vi "FPGA_fast cycles-4.vi"() -> ()   [LabVIEW 2013]
uses:
  fast cycles/FPGA_run-states.ctl
  <vilib>/rvi/Emulation/niFpgaSctlEmulationGetInTimedLoop.vi
  <vilib>/rvi/Emulation/niFpgaEmulationReportErrorSimple.vi
  <vilib>/rvi/Emulation/niFpgaGetClockAttributes.vi
  <vilib>/rvi/FIFO/Fifo_Resource/nirvififoEmulationReadFpgaImpl.vi
  <vilib>/rvi/DataTransferAndStorage/Container/Common/niFpgaContainerGetUniqueNameForEmu.vi
  <vilib>/rvi/Emulation/niFpgaProcessEmulError.vi
  <vilib>/rvi/Memory/Memory_Emulation/nirvimemoryEmulation.vi
  <vilib>/rvi/Memory/Memory_Emulation/nirvimemoryFastEmulation.vi
  <vilib>/rvi/Memory/Memory_Emulation/niFpgaMemoryEmulationCacheClearOnFirstRun.vi
  <vilib>/rvi/Memory/Memory_Emulation/nirvimemoryEmulationManagerCache_MakeExclusive.vi
  <vilib>/rvi/Memory/Memory_Emulation/niFpgaMemoryEmulationValidateCache.vi
  <vilib>/rvi/Memory/Memory_Emulation/nirvimemoryEmulationManagerCache_ReleaseExclusive.vi
  <vilib>/rvi/Memory/Memory_Emulation/nirvimemoryEmulationManagerCache_InsertValue.vi
  <vilib>/Utility/error.llb/Clear Errors.vi
  <vilib>/rvi/Memory/Memory_Emulation/nirvimemoryEmulationManagerCache_SetValue.vi
  <vilib>/rvi/Emulation/niFpgaSctlEmulationResourceMgr.vi
  <vilib>/rvi/Emulation/niFpgaCriticalErrorInLSC.vi
  <vilib>/rvi/Memory/Memory_Emulation/nirvimemoryEmulationManagerCache_GetValue.vi
  <vilib>/rvi/FIFO/Fifo_Resource/nirvififoEmulationWriteFpgaImpl.vi
  <vilib>/rvi/eio/common/nirviEmuTemplateMethod_errors.vi
  <vilib>/rvi/DataTransferAndStorage/Container/XNode/niFpgaContainer.xnode
  <vilib>/rvi/FIFO/Fifo_Resource/nirvififoEmulationRead.vi
  <vilib>/rvi/FIFO/Fifo_Resource/nirvififoEmulationWrite.vi
  <vilib>/eio/EIONode/EIONode.xnode
panel:
  out "ramp":bool
  out "trigDAC":bool
  in  "order in":u64=360850920143060992
  in  "get order":bool
  in  "Stop seq 2":bool=TRUE
  in  "stop on sample count":bool
  in  "samples":u16=1
  in  "pulse length":u16=100
  in  "Divider":u32=200000
  out "voltmeters trig":bool=TRUE
  in  "Stop seq":bool=TRUE
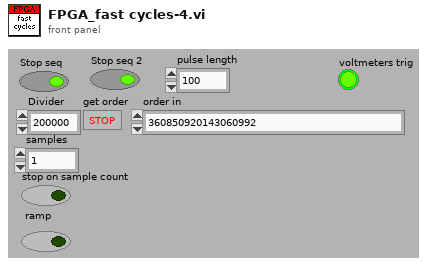
[diagram p1: front panel]
types:
  T1 = typedef "FPGA_run-states.ctl" = enum16{"stopped", "check", "reserve", "run", "release"}
  T2 = cluster{"Boolean array[0]":bool, "Boolean array[1]":bool, "Boolean array[2]":bool, "Boolean array[3]":bool, "Boolean array[4]":bool, "Boolean array[5]":bool, "Boolean array[6]":bool, "Boolean array[7]":bool, "Boolean array[8]":bool, "Boolean array[9]":bool, "Boolean array[10]":bool, "Boolean array[11]":bool, "Boolean array[12]":bool, "Boolean array[13]":bool, "Boolean array[14]":bool, "Boolean array[15]":bool}
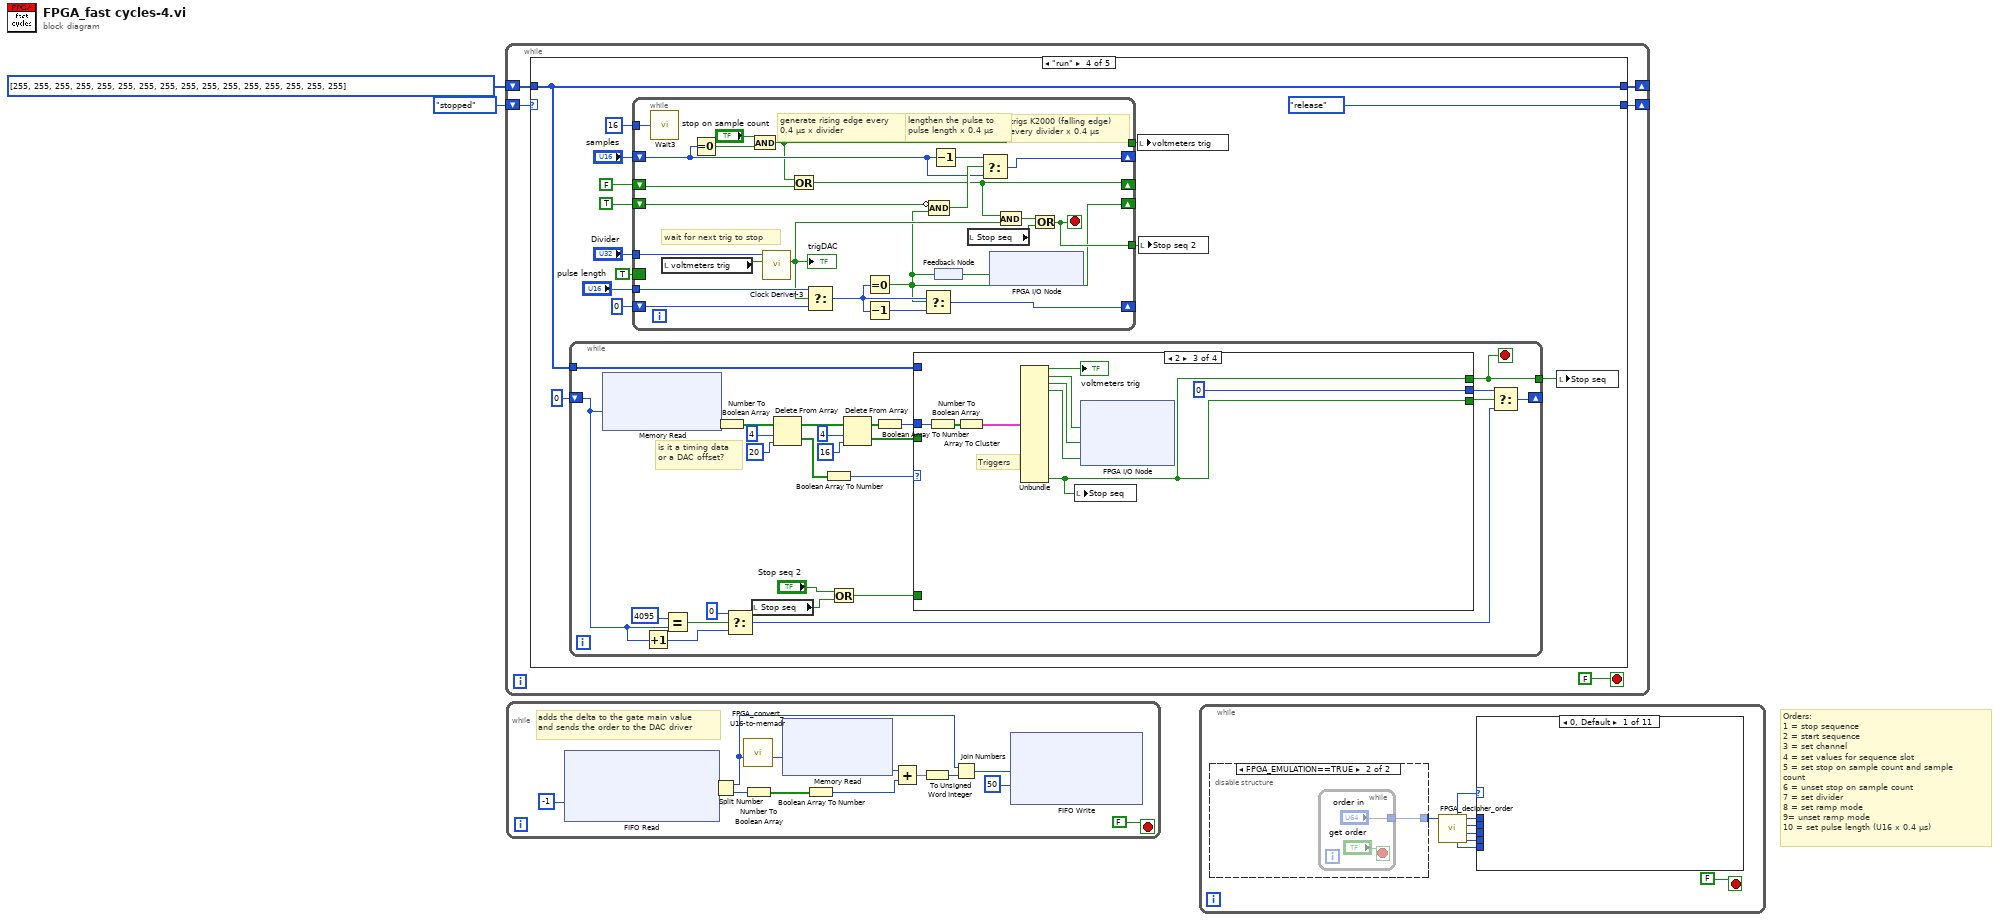
[diagram p0: block diagram]
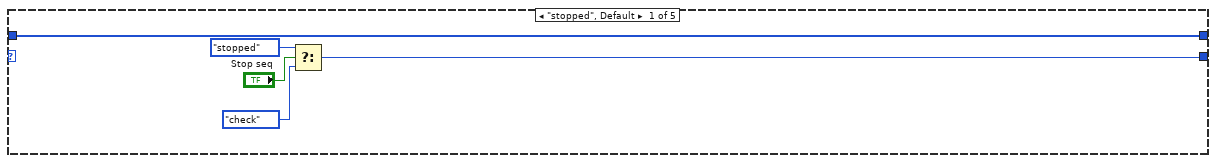
[diagram p2: hidden frame]
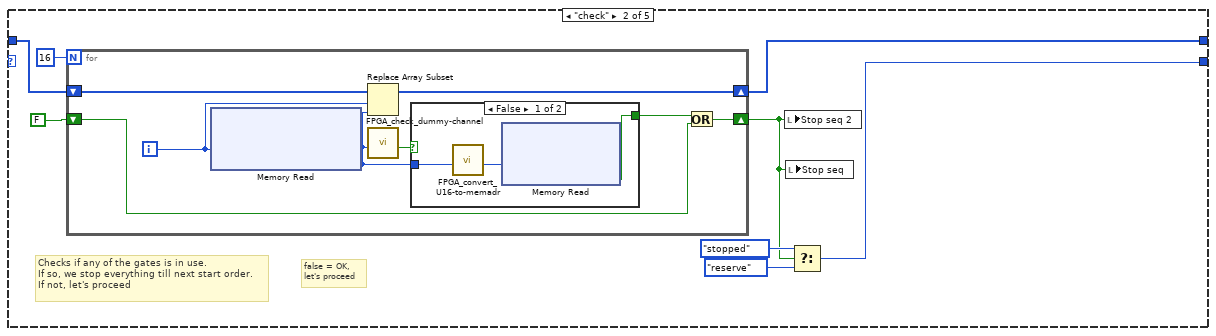
[diagram p3: hidden frame]
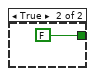
[diagram p4: hidden frame]
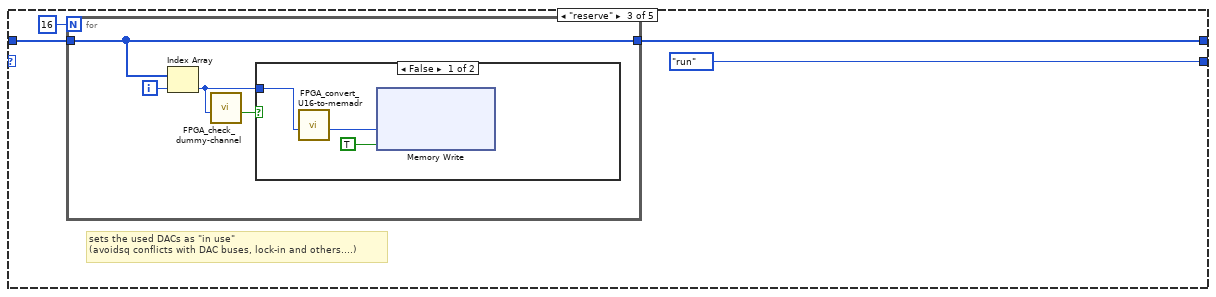
[diagram p5: hidden frame]
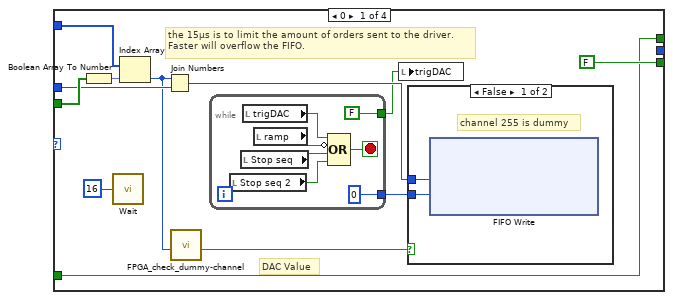
[diagram p7: hidden frame]
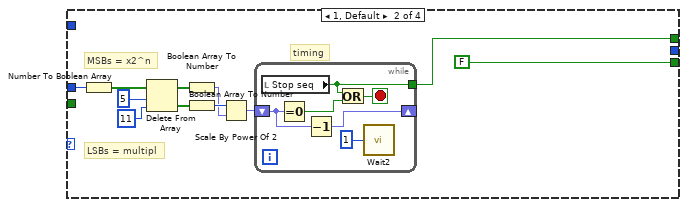
[diagram p9: hidden frame]
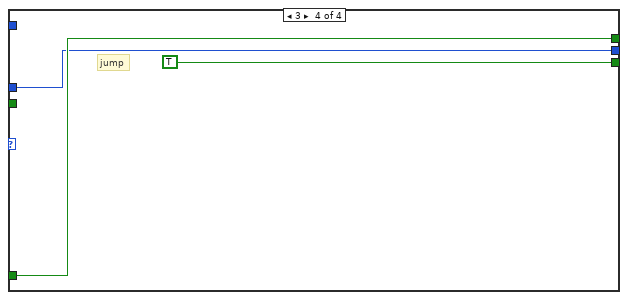
[diagram p10: hidden frame]
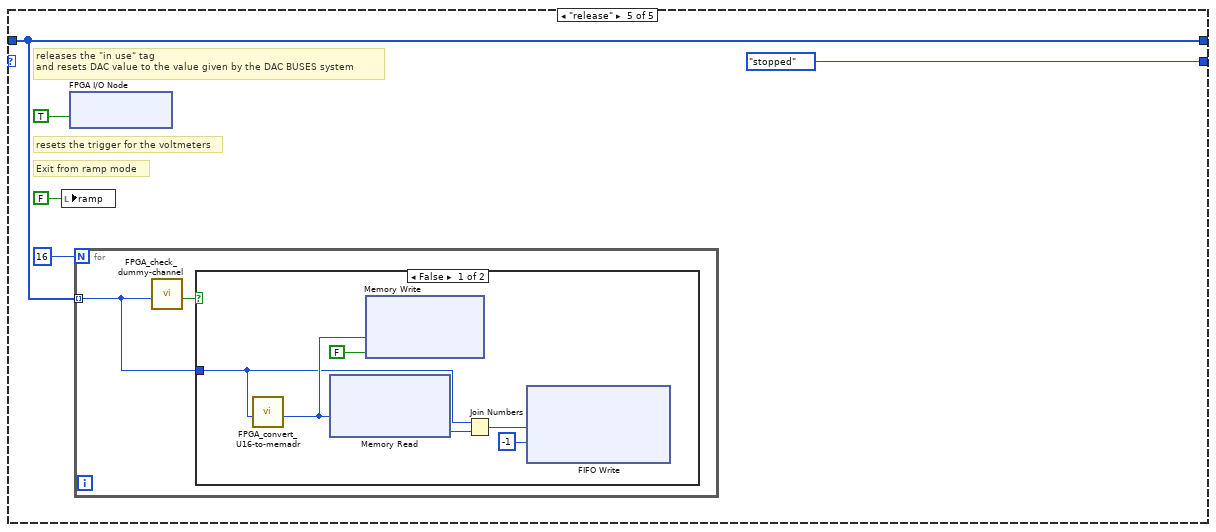
[diagram p11: hidden frame]
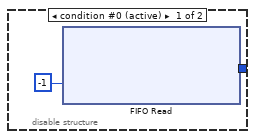
[diagram p13: hidden frame]
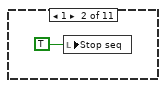
[diagram p14: hidden frame]
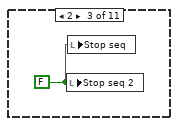
[diagram p15: hidden frame]
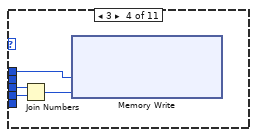
[diagram p16: hidden frame]
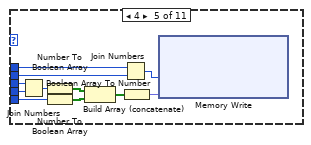
[diagram p17: hidden frame]
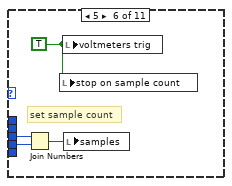
[diagram p18: hidden frame]
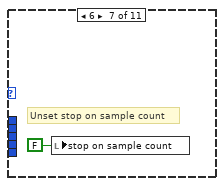
[diagram p19: hidden frame]
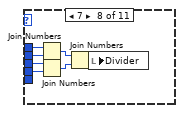
[diagram p20: hidden frame]
diagram:
  # "Orders:\n1 = stop sequence\n2 = start sequence\n3 = set channel\n4 = set values for sequence slot\n5 = set stop on sample count and sample count\n6 = unset stop on sample count\n7 = set divider\n8 = set ramp mode\n9= unset ramp mode\n10 = set pulse length (U16 x 0.4 µs)"
  n1 = while {
    shift-right: [w5] -> _
    shift-left: FPGA_run-states."stopped" ("run states") -> [w6]
    shift-right: [w3] -> _
    shift-left: u16[] [255, 255, 255, 255, 255, 255, 255, 255, 255, 255, 255, 255, 255, 255, 255, 255] -> [w4]
    stop <- FALSE stop-if-true
    n2 = case shown="\"run\"" w6 {
      tunnel: [w9 w13 FPGA_run-states."run" ("run states") FPGA_run-states."release" ("run states") FPGA_run-states."stopped" ("run states")] -> w5
      tunnel: [w8 w14 w33 w47 w159] -> w3
      tunnel: w4 -> [w8 w15 w34 w47 w159]
      frame "stopped", Default {
        n3 = Select(t=FPGA_run-states."stopped" ("run states"), s="Stop seq", f=FPGA_run-states."check" ("run states")) -> (s? t:f=w9:T1)
      }
      frame "check" {
        # "Checks if any of the gates is in use.\nIf so, we stop everything till next start order.\nIf not, let's proceed"
        # "false = OK,\nlet's proceed"
        n4 = for {
          N: 16 -> [_]
          shift-right: [w26] -> w16
          shift-left: FALSE ("Data") -> [w25]
          shift-right: [w24] -> w14
          shift-left: w15 -> [w23]
          i -> [w28]
          n5 = xnode ("Memory Read")("Address"=w28) -> ("Data"=w21:u16)  [unwired: 1 in, 1 out]
          n6 = Replace Array Subset(array=w23, new element=w21, index=w28) -> (w24:u16[])
          n7 = call "FPGA_check_dummy-channel.vi"("pan-channel"=w21) -> ("dummy?"=w22:bool)  [unwired: 10 out]
          n8 = case shown="False" w22 {
            tunnel: w21 -> [w31 _]
            tunnel: [w29 FALSE ("Data")] -> w27
            frame False {
              n9 = call "FPGA_convert_U16-to-memadr.vi"("Numeric"=w31) -> ("mem adr"=w30:u8)  [unwired: 10 out]
              n10 = xnode ("Memory Read")("Address"=w30) -> ("Data"=w29:bool)  [unwired: 1 in, 1 out]
            }
            frame True {
            }
          }
          n11 = Or(x=w27, y=w25) -> (x .or. y?=w26:bool)
        }
        n12 = local write "Stop seq 2"(w16) -> ()
        n13 = local write "Stop seq"(w16) -> ()
        n14 = Select(t=FPGA_run-states."stopped" ("run states"), s=w16, f=FPGA_run-states."reserve" ("run states")) -> (s? t:f=w13:T1)
      }
      frame "reserve" {
        # "sets the used DACs as \"in use\"\n(avoidsq conflicts with DAC buses, lock-in and others....)"
        n15 = for {
          N: 16 -> [_]
          tunnel: w34 -> [w39]
          tunnel: [w39] -> w33
          i -> [w40]
          n16 = Index Array(array=w39, index=w40) -> (element=w38:u16)
          n17 = call "FPGA_check_dummy-channel.vi"("pan-channel"=w38) -> ("dummy?"=w37:bool)  [unwired: 10 out]
          n18 = case shown="False" w37 {
            tunnel: w38 -> [w41 _]
            frame False {
              n19 = call "FPGA_convert_U16-to-memadr.vi"("Numeric"=w41) -> ("mem adr"=w43:u8)  [unwired: 10 out]
              n20 = xnode ("Memory Write")("Address"=w43, "Data"=TRUE) -> ()  [unwired: 1 in, 1 out]
            }
            frame True {
            }
          }
        }
      }
      frame "run" {
        n21 = while {
          shift-right: [w90] -> _
          shift-left: u16 0 ("t") -> [w102]
          tunnel: [w83] -> w49
          tunnel: w47 -> [w82]
          stop <- w83 stop-if-true
          # "is it a timing data\nor a DAC offset?"
          n22 = xnode ("Memory Read")("Address"=w102) -> ("Data"=w101:fxp<+,24,24>)  [unwired: 1 in, 1 out]
          n23 = Increment(x=w102) -> (x+1=w104:u16)
          n24 = Equal?(x=u16 4095, y=w102) -> (x = y?=w106:bool)
          n25 = Number To Boolean Array(number=w101) -> (Boolean array=w100:bool[])
          n26 = Select(t=u16 0, s=w106, f=w104) -> (s? t:f=w103:u16)
          n27 = local read "Stop seq"() -> (w87:bool)
          n28 = Delete From Array(array=w100, length=4, index=20) -> (deleted portion=w93:bool[], array with subset deleted=w97:bool[])
          n29 = Boolean Array To Number(Boolean array=w93) -> (number=w91:u8)
          n30 = Or(x="Stop seq 2", y=w87) -> (x .or. y?=w85:bool)
          n31 = Delete From Array(array=w97, length=4, index=16) -> (deleted portion=w94:bool[], array with subset deleted=w95:bool[])
          n32 = Boolean Array To Number(Boolean array=w95) -> (number=w86:u16)
          n33 = case shown="2" w91 {
            tunnel: w86 -> [w117 w139 w154 w155]
            tunnel: w94 -> [w119 _ _ _]
            tunnel: [FALSE ("Stop seq") FALSE ("Stop seq") w148 TRUE ("Stop seq")] -> w89
            tunnel: [_ _ u16 0 w155] -> w88
            tunnel: [w113 w129 w148 w156] -> w83
            tunnel: w85 -> [w113 _ _ w156]
            tunnel: w82 -> [w111 _ _ _]
            frame 0 {
              # "the 15µs is to limit the amount of orders sent to the driver.\nFaster will overflow the FIFO."
              # "DAC Value"
              n34 = Boolean Array To Number(Boolean array=w119) -> (number=w118:fxp<+,4,4>)
              n35 = call "Wait"("Count(uSec)"=u8 16) -> ()  [unwired: 1 out]
              n36 = Index Array(array=w111, index=w118) -> (element=w109:u16)
              n37 = Join Numbers(hi=w109, lo=w117) -> ((hi.lo)=w116:u32)
              n38 = call "FPGA_check_dummy-channel.vi"("pan-channel"=w109) -> ("dummy?"=w110:bool)  [unwired: 10 out]
              n39 = while {
                tunnel: [0 ("Timeout")] -> w112
                tunnel: [FALSE ("Stop seq 3")] -> w108
                stop <- w123 stop-if-true
                n40 = local read "Stop seq 2"() -> (w126:bool)
                n41 = local read "Stop seq"() -> (w127:bool)
                n42 = local read "trigDAC"() -> (w124:bool)
                n43 = local read "ramp"() -> (w125:bool)
                n44 = Compound Arithmetic op=OR(w124, invert w125, w127, w126) -> (w123:bool)
              }
              n45 = local write "trigDAC"(w108) -> ()
              n46 = case shown="False" w110 {
                tunnel: w116 -> [w121 _]
                tunnel: w112 -> [w120 _]
                frame False {
                  # "channel 255 is dummy"
                  n47 = xnode ("FIFO Write")("Element"=w121, "Timeout"=w120) -> ()  [unwired: 1 in, 2 out]
                }
                frame True {
                }
              }
            }
            frame 1, Default {
              # "MSBs = x2^n"
              # "LSBs = multipl"
              # "timing"
              n48 = Number To Boolean Array(number=w139) -> (Boolean array=w138:bool[])
              n49 = Delete From Array(array=w138, length=5 ("longueur"), index=11 ("indice")) -> (deleted portion=w134:bool[], array with subset deleted=w135:bool[])
              n50 = Boolean Array To Number ("Tableau de booléens en nombre")(Boolean array=w135) -> (number=w132:fxp<+,37,37>)
              n51 = Boolean Array To Number ("Tableau de booléens en nombre")(Boolean array=w134) -> (number=w133:u8)
              n52 = Scale By Power Of 2(n=w133, x=w132) -> (x*2^n=w131:fxp<+,37,37>)
              n53 = while {
                shift-right: [w145] -> _
                shift-left: w131 -> [w144]
                tunnel: [w140] -> w129
                stop <- w143 stop-if-true
                n54 = local read "Stop seq"() -> (w140:bool)
                n55 = Equal To 0?(x=w144) -> (x = 0?=w141:bool)
                n56 = Decrement ("Décrémenter")(x=w144) -> (x-1=w145:fxp<+,37,37>)
                n57 = Or(x=w140, y=w141) -> (x .or. y?=w143:bool)
                n58 = call "Wait2"("Count(uSec)"=u8 1) -> ()  [unwired: 1 out]
              }
            }
            frame 2 {
              # "Triggers"
              n59 = Number To Boolean Array(number=w154) -> (Boolean array=w153:bool[])
              n60 = Array To Cluster(array=w153) -> (cluster=w152:T2)
              n61 = Unbundle(w152) -> ("Boolean array[0]"=→"voltmeters trig":bool, "Boolean array[1]"=w151:bool, "Boolean array[2]"=w150:bool, "Boolean array[3]"=w147:bool, "Boolean array[15]"=w148:bool)  [unwired: 11 out]
              n62 = local write "Stop seq"(w148) -> ()
              n63 = xnode "FPGA I/O Node"("Port0/DIO2"=w151, "Port0/DIO3"=w150, "Port0/DIO4"=w147) -> ()  [unwired: 3 in, 3 out]
            }
            frame 3 {
              # "jump"
            }
          }
          n64 = Select(t=w88, s=w89, f=w103) -> (s? t:f=w90:u16)
        }
        n65 = while {
          tunnel: "Divider" -> [w81]
          tunnel: "pulse length" -> [w79]
          shift-right: [w76] -> _
          shift-left: u16 0 ("pulse length") -> [w78]
          shift-right: [w73] -> _
          shift-left: "samples" -> [w72]
          shift-right: [w58] -> _
          shift-left: TRUE -> [w59]
          tunnel: u8 16 ("Count(Ticks)") -> [w71]
          tunnel: [w67] -> w51
          tunnel: [w68] -> w50
          shift-right: [w63] -> _
          shift-left: FALSE -> [w65]
          border: TRUE -> [_]
          stop <- w68 stop-if-true
          # "wait for next trig to stop"
          # "trigs K2000 (falling edge)\nevery divider x 0.4 µs"
          # "lengthen the pulse to\npulse length x 0.4 µs"
          # "generate rising edge every\n0.4 µs x divider"
          n66 = call "Wait3"("Count(Ticks)"=w71) -> ()  [unwired: 1 out]
          n67 = local read "voltmeters trig"() -> (w69:bool)
          n68 = Equal To 0?(x=w72) -> (x = 0?=w61:bool)
          n69 = And(x="stop on sample count", y=w61) -> (x .and. y?=w67:bool)
          n70 = call "Clock Deriver-3.vi"("reset"=w69, "Divisor"=w81) -> ("Clock Out"=w62:bool)  [unwired: 1 in, 8 out]
          "trigDAC" <- w62
          n71 = Or(x=w67, y=w65) -> (x .or. y?=w63:bool)
          n72 = Select(t=w79, s=w62, f=w78) -> (s? t:f=w77:u16)
          n73 = Equal To 0?(x=w77) -> (x = 0?=w58:bool)
          n74 = Decrement(x=w77) -> (x-1=w80:u16)
          n75 = Select(t=w77, s=w58, f=w80) -> (s? t:f=w76:u16)
          n76 = Compound Arithmetic op=AND(invert w59, w58) -> (w75:bool)
          n77 = Decrement(x=w72) -> (x-1=w74:u16)
          n78 = feedback-in #1(w58) -> ()
          n79 = feedback #1() -> (w64:bool)
          n80 = local read "Stop seq"() -> (w70:bool)
          n81 = Select(t=w74, s=w75, f=w72) -> (s? t:f=w73:u16)
          n82 = xnode "FPGA I/O Node"("Port0/DIO1"=w64) -> ()  [unwired: 1 in, 1 out]
          n83 = And(x=w63, y=w62) -> (x .and. y?=w66:bool)
          n84 = Or(x=w66, y=w70) -> (x .or. y?=w68:bool)
        }
        n85 = local write "voltmeters trig"(w51) -> ()
        n86 = local write "Stop seq 2"(w50) -> ()
        n87 = local write "Stop seq"(w49) -> ()
      }
      frame "release" {
        # "Exit from ramp mode"
        # "resets the trigger for the voltmeters"
        # "releases the \"in use\" tag\nand resets DAC value to the value given by the DAC BUSES system"
        n88 = local write "ramp"(FALSE ("ramp")) -> ()
        n89 = xnode "FPGA I/O Node"("Port0/DIO1"=TRUE ("Port9/DIO1")) -> ()  [unwired: 1 in, 1 out]
        n90 = for {
          N: 16 -> [_]
          tunnel: w159 -> [w163] mode=indexing
          n91 = call "FPGA_check_dummy-channel.vi"("pan-channel"=w163) -> ("dummy?"=w164:bool)  [unwired: 10 out]
          n92 = case shown="False" w164 {
            tunnel: w163 -> [w165 _]
            frame False {
              n93 = call "FPGA_convert_U16-to-memadr.vi"("Numeric"=w165) -> ("mem adr"=w169:u8)  [unwired: 10 out]
              n94 = xnode ("Memory Read")("Address"=w169) -> ("Data"=w167:u16)  [unwired: 1 in, 1 out]
              n95 = xnode ("Memory Write")("Address"=w169, "Data"=FALSE) -> ()  [unwired: 1 in, 1 out]
              n96 = Join Numbers(hi=w165, lo=w167) -> ((hi.lo)=w168:u32)
              n97 = xnode ("FIFO Write")("Element"=w168, "Timeout"=-1) -> ()  [unwired: 1 in, 2 out]
            }
            frame True {
            }
          }
        }
      }
    }
  }
  n98 = while {
    stop <- FALSE stop-if-true
    # "adds the delta to the gate main value\nand sends the order to the DAC driver"
    n99 = xnode ("FIFO Read")("Timeout"=-1) -> ("Element"=w182:u32)  [unwired: 1 in, 2 out]
    n100 = Split Number(x=w182) -> (hi(x)=w172:u16, lo(x)=w174:u16)
    n101 = call "FPGA_convert_U16-to-memadr.vi"("Numeric"=w172) -> ("mem adr"=w173:u8)  [unwired: 10 out]
    n102 = Number To Boolean Array(number=w174) -> (Boolean array=w179:bool[])
    n103 = xnode ("Memory Read")("Address"=w173) -> ("Data"=w181:u16)  [unwired: 1 in, 1 out]
    n104 = Boolean Array To Number(Boolean array=w179) -> (number=w178:i16)
    n105 = Add(x=w181, y=w178) -> (x+y=w177:fxp<+,16,16>)
    n106 = To Unsigned Word Integer(number=w177) -> (unsigned 16bit integer=w175:u16)
    n107 = Join Numbers(hi=w172, lo=w175) -> ((hi.lo)=w176:u32)
    n108 = xnode ("FIFO Write")("Element"=w176, "Timeout"=50) -> ()  [unwired: 1 in, 2 out]
  }
  n109 = while {
    stop <- FALSE stop-if-true
    n110 = disable-structure shown="FPGA_EMULATION==TRUE" {
      disable-tunnel: [w192 w194] -> w190
      frame condition #0 (active) {
        n111 = xnode ("FIFO Read")("Timeout"=-1) -> ("Element"=w192:u64)  [unwired: 1 in, 2 out]
      }
      frame condition #1 {
        n112 = while {
          tunnel: ["order in"] -> w194
          stop <- "get order" stop-if-true
        }
      }
    }
    n113 = call "FPGA_decipher_order.vi"("order in"=w190) -> ("data 1"=w188:u8, "data 2"=w187:u8, "data 3"=w185:u8, "data 4"=w186:u8, "RFU 2"=w184:u8, "order out"=w189:u8)  [unwired: 5 out]
    n114 = case shown="0, Default" w189 {
      tunnel: w188 -> [_ _ _ w200 w213 w216 _ w222 w228 _ w234]
      tunnel: w187 -> [_ _ _ w201 w212 w217 _ w223 w227 _ w233]
      tunnel: w186 -> [_ _ _ w202 w206 _ _ w225 _ _ _]
      tunnel: w185 -> [_ _ _ _ w205 _ _ w224 _ _ _]
      tunnel: w184 -> [_ _ _ _ w203 _ _ _ _ _ _]
      frame 0, Default {
      }
      frame 1 {
        n115 = local write "Stop seq"(TRUE ("Stop seq")) -> ()
      }
      frame 2 {
        w198 = FALSE ("Stop seq")
        n116 = local write "Stop seq 2"(w198) -> ()
        n117 = local write "Stop seq"(w198) -> ()
      }
      frame 3 {
        n118 = Join Numbers(hi=w201, lo=w200) -> ((hi.lo)=w199:u16)
        n119 = xnode ("Memory Write")("Address"=w202, "Data"=w199) -> ()  [unwired: 1 in, 1 out]
      }
      frame 4 {
        n120 = Join Numbers(hi=w212, lo=w213) -> ((hi.lo)=w211:u16)
        n121 = Number To Boolean Array(number=w211) -> (Boolean array=w210:bool[])
        n122 = Number To Boolean Array(number=w203) -> (Boolean array=w209:bool[])
        n123 = Build Array (concatenate)(w210, w209) -> (w208:bool[])
        n124 = Join Numbers(hi=w206, lo=w205) -> ((hi.lo)=w207:u16)
        n125 = Boolean Array To Number(Boolean array=w208) -> (number=w204:fxp<+,24,24>)
        n126 = xnode ("Memory Write")("Address"=w207, "Data"=w204) -> ()  [unwired: 1 in, 1 out]
      }
      frame 5 {
        w214 = TRUE
        # "set sample count"
        n127 = Join Numbers(hi=w217, lo=w216) -> ((hi.lo)=w215:u16)
        n128 = local write "stop on sample count"(w214) -> ()
        n129 = local write "voltmeters trig"(w214) -> ()
        n130 = local write "samples"(w215) -> ()
      }
      frame 6 {
        # "Unset stop on sample count"
        n131 = local write "stop on sample count"(FALSE) -> ()
      }
      frame 7 {
        n132 = Join Numbers(hi=w225, lo=w224) -> ((hi.lo)=w221:u16)
        n133 = Join Numbers(hi=w223, lo=w222) -> ((hi.lo)=w220:u16)
        n134 = Join Numbers(hi=w221, lo=w220) -> ((hi.lo)=w219:u32)
        n135 = local write "Divider"(w219) -> ()
      }
      frame 8 {
        w230 = TRUE
        n136 = Join Numbers(hi=w227, lo=w228) -> ((hi.lo)=w229:u16)
        n137 = local write "stop on sample count"(w230) -> ()
        n138 = local write "trigDAC"(FALSE ("trigDAC")) -> ()
        n139 = local write "voltmeters trig"(w230) -> ()
        n140 = local write "samples"(w229) -> ()
        "ramp" <- w230
      }
      frame 9 {
        w231 = FALSE
        n141 = local write "stop on sample count"(w231) -> ()
        n142 = local write "ramp"(w231) -> ()
      }
      frame 10 {
        # "set the length of"
        n143 = Join Numbers(hi=w233, lo=w234) -> ((hi.lo)=w232:u16)
        n144 = local write "pulse length"(w232) -> ()
      }
    }
  }
